vi "Bildcluster.vi"(6 "Build Specification Version":T1, 8 "error in (no error)":errorcluster, 9 "BuildItem":T2, 10 "path":path, 11 "String in":refnum<vi>) -> (0 "error out":errorcluster)   [LabVIEW 2017]
uses:
  BuildItem.ctl
  <vilib>/AppBuilder/AB_API_Simple/Build Specification Version.ctl
  <vilib>/AppBuilder/AB_API_Simple/NI_App_Builder_API.lvlib
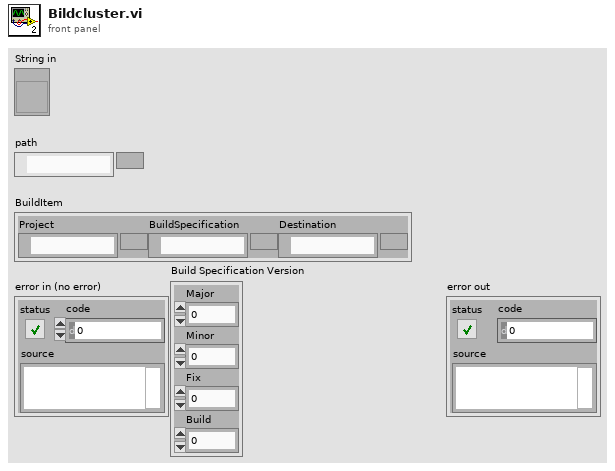
[diagram p1: front panel]
types:
  T1 = typedef "NI_App_Builder_API.lvlib/Build Specification Version.ctl" = cluster{"Major":u16, "Minor":u16, "Fix":u16, "Build":u16}
  T2 = typedef "BuildItem.ctl" = cluster{"Project":path, "BuildSpecification":path, "Destination":path}
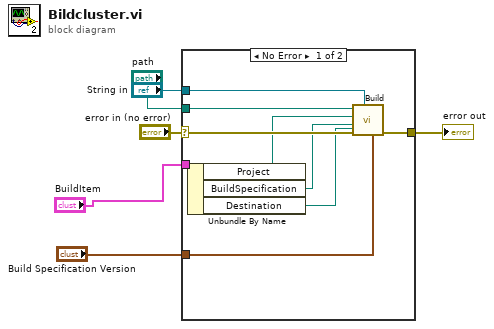
[diagram p0: block diagram]
diagram:
  n1 = case shown="No Error" "error in (no error)" {
    selector: "error in (no error)" -> [w12 w16]
    tunnel: "BuildItem" -> [w11 _]
    tunnel: "String in" -> [w15 _]
    tunnel: "path" -> [w14 _]
    tunnel: [w13 w16] -> w4
    tunnel: "Build Specification Version" -> [w7 _]
    frame No Error {
      n2 = Unbundle By Name(w11) -> ("Project"=w10:path, "BuildSpecification"=w9:path, "Destination"=w8:path)
      n3 = call "Build.vi"("Build Specification Version"=w7, "Destination"=w8, "String in"=w15, "error in"=w12, "BuildSpecification"=w9, "Project"=w10, "WorkspaceFolder"=w14) -> ("error out"=w13:errorcluster)  [unwired: 4 in]
    }
    frame Error {
    }
  }
  "error out" <- w4
